vi "IsOperationSuccessful.vi"(8 "error in (no error)":errorcluster, 11 "Generated files":path[](array[path])) -> (0 "error out":errorcluster, 2 "Is Successful?":bool, 3 "Output/Failure message":string)   [LabVIEW 2014, in "ExecuteBuildSpec.lvclass"]
uses:
  ExecuteBuildSpec.lvclass
panel:
  in  "Failure message":string="ExecuteBuildSpec operation failed. No files were generated."
  in  "Output message":string="Generated files are:\\n%s"
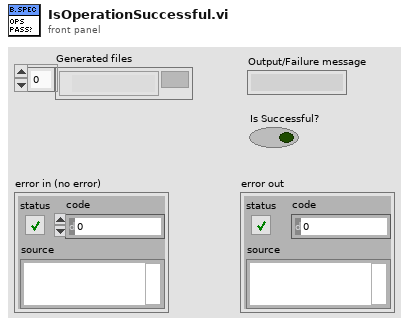
[diagram p1: front panel]
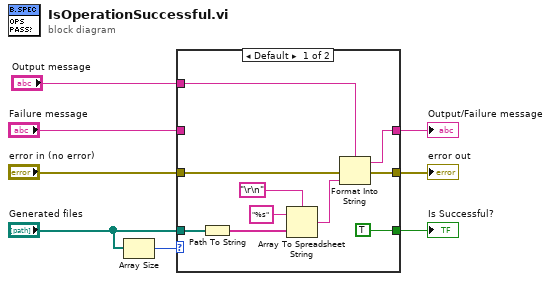
[diagram p0: block diagram]
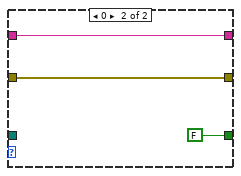
[diagram p2: hidden frame]
diagram:
  n1 = Array Size(array="Generated files") -> (size(s)=w3:i32)
  n2 = case shown="Default" w3 {
    tunnel: "Generated files" -> [w17 _]
    tunnel: [TRUE FALSE] -> w5
    tunnel: [w13 w19] -> w6
    tunnel: "error in (no error)" -> [w12 w20]
    tunnel: [w11 w20] -> w8
    tunnel: "Output message" -> [w10 _]
    tunnel: "Failure message" -> [_ w19]
    frame Default {
      n3 = Path To String(path=w17) -> (string=w16:string[])
      n4 = Array To Spreadsheet String(delimiter (Tab)="\r\n", array=w16, 3:"%s" ("format string")) -> (spreadsheet string=w14:string)
      n5 = Format Into String(format string=w10, error in=w12, w14) -> (resulting string=w13:string, error out=w11:errorcluster)  [unwired: 1 in]
    }
    frame 0 {
    }
  }
  "error out" <- w8
  "Output/Failure message" <- w6
  "Is Successful?" <- w5
